vi "step.vi"(8 "error in (no error)":errorcluster, 10 "pStmt":i64, 11 "psqlite":refnum<class "sqlite3.lvclass">) -> (0 "error out":errorcluster, 3 "finished?":bool)   [LabVIEW 2014, in "SQLite3LV.lvlib" / "cursor.lvclass"]
uses:
  cursor.lvclass
  SQLite3 Class/sqlite3.lvclass
  SQLite3LV.lvlib
  sqlite3_64.dll
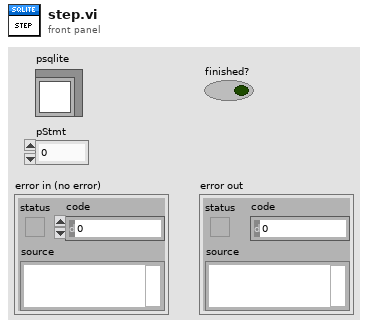
[diagram p1: front panel]
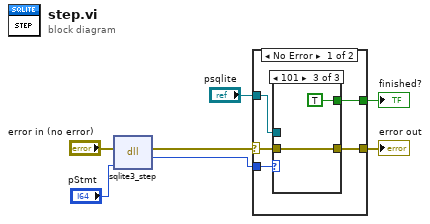
[diagram p0: block diagram]
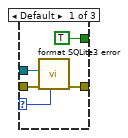
[diagram p2: hidden frame]
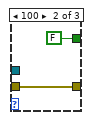
[diagram p3: hidden frame]
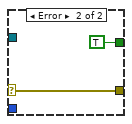
[diagram p4: hidden frame]
diagram:
  n1 = dll-call lib="C:/Users/BobUser/Desktop/LVTables/sqlite3**.*" fn="sqlite3_step"(error in="error in (no error)", "pStmt"="pStmt") -> (error out=w3:errorcluster, "result"=w4:i32)  [unwired: 3 in, 1 out]
  n2 = case shown="No Error" w3 {
    selector: w3 -> [w11 w23]
    tunnel: w4 -> [w12 _]
    tunnel: [w10 w23] -> w5
    tunnel: [w9 TRUE] -> w6
    tunnel: "psqlite" -> [w8 _]
    frame No Error {
      n3 = case shown="101" w12 {
        selector: w12 -> [w16 _ _]
        tunnel: w11 -> [w17 w18 w20]
        tunnel: [w15 w18 w20] -> w10
        tunnel: [TRUE FALSE TRUE] -> w9
        tunnel: w8 -> [w13 _ _]
        frame Default {
          n4 = call "format SQLite3 error.vi"("SQLite3LV Connection result"=w16, "error in (no error)"=w17, "psqlite"=w13) -> ("error out"=w15:errorcluster)  [unwired: 8 in]
        }
        frame 100 {
        }
        frame 101 {
        }
      }
    }
    frame Error {
    }
  }
  "finished?" <- w6
  "error out" <- w5
